vi "Edgertronic-get_camstatus.vi"(3 "error in (no error)":errorcluster, 5 "URL":string="192.168.1.101") -> (0 "error out":errorcluster, 1 "Cam Status":T2={"Level"="20140911165611", "Flags"="20140911165611", "Is Temp"="20140911165611", "FPGA Temp"="20140911165611", "State"="20140911165611", "Camera Time"="20140911165611", "dacvrefadc"="20140911165611", "Connection Information:"=""}, 2 "Status":T1={"Pretrigger Fill Level"=0, "IS Temp"=0.0, "State"=0, "dacvrefadc"="20140911165611", "Flags"={"Storage full"=FALSE, "Storage missing"=FALSE, "USB Storage installed"=FALSE, "SD Card installed"=FALSE, "USB full"=FALSE, "SD Card full"=FALSE, "Bad storage"=FALSE, "Net Configured"=FALSE, "Net unmountable"=FALSE, "Net full"=FALSE, "Storage full 11"=FALSE, "Storage full 12"=FALSE, "Storage full 13"=FALSE, "Storage full 14"=FALSE, "Storage full 15"=FALSE, "Storage full 16"=FALSE, "Storage full 17"=FALSE, "Genlock - no signal"=FALSE, "Genlock - config err"=FALSE}, "FPGA Temp"=0.0, "Camera time"=timestamp(0 s since 1904-01-01)} {"FPGA Temp" scale=0.0..100.0; "State" items=["Unconfigured", "Calibrating", "Running", "Triggered", "Saving", "Pretrigger full", "Trigger Canceled", "Save Canceled"]; "IS Temp" scale=0.0..100.0; "Pretrigger Fill Level" scale=0.0..100.0})   [LabVIEW 2015]
doc: "This VI returns the camera status information."
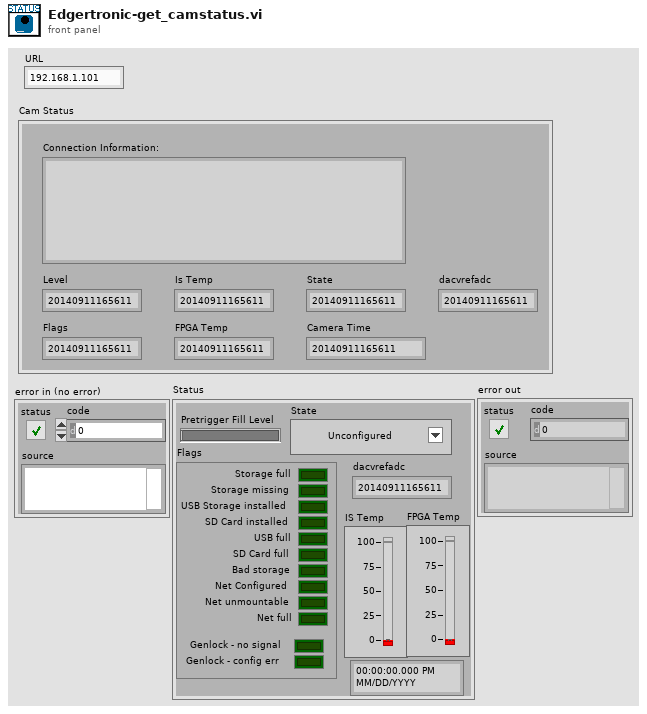
[diagram p1: front panel]
types:
  T1 = cluster{"Pretrigger Fill Level":u8, "IS Temp":dbl, "State":u16, "dacvrefadc":string, "Flags":cluster{"Storage full":bool, "Storage missing":bool, "USB Storage installed":bool, "SD Card installed":bool, "USB full":bool, "SD Card full":bool, "Bad storage":bool, "Net Configured":bool, "Net unmountable":bool, "Net full":bool, "Storage full 11":bool, "Storage full 12":bool, "Storage full 13":bool, "Storage full 14":bool, "Storage full 15":bool, "Storage full 16":bool, "Storage full 17":bool, "Genlock - no signal":bool, "Genlock - config err":bool}, "FPGA Temp":dbl, "Camera time":timestamp}
  T2 = cluster{"Level":string, "Flags":string, "Is Temp":string, "FPGA Temp":string, "State":string, "Camera Time":string, "dacvrefadc":string, "Connection Information:":string}
  T3 = cluster{"Boolean array[0]":bool, "Boolean array[1]":bool, "Boolean array[2]":bool, "Boolean array[3]":bool, "Boolean array[4]":bool, "Boolean array[5]":bool, "Boolean array[6]":bool, "Boolean array[7]":bool, "Boolean array[8]":bool, "Boolean array[9]":bool, "Boolean array[10]":bool, "Boolean array[11]":bool, "Boolean array[12]":bool, "Boolean array[13]":bool, "Boolean array[14]":bool, "Boolean array[15]":bool, "Boolean array[16]":bool, "Boolean array[17]":bool, "Boolean array[18]":bool}
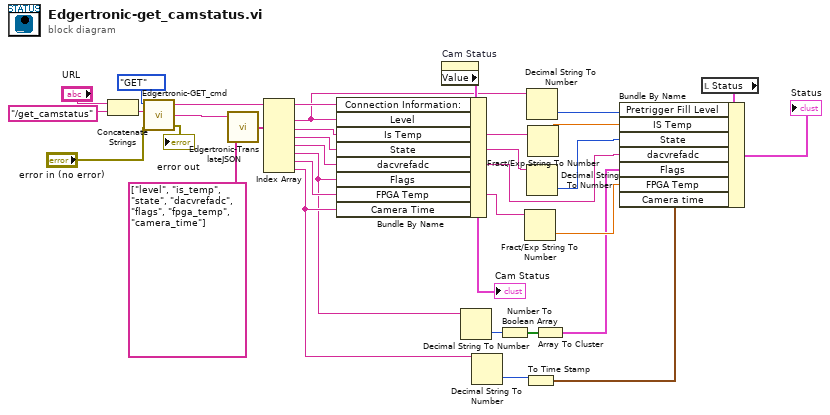
[diagram p0: block diagram]
diagram:
  n1 = Concatenate Strings("URL", "/get_camstatus" ("GET Cmd")) -> (w3:string)
  n2 = call "Edgertronic-GET_cmd.vi"("error in (no error)"="error in (no error)", "URL"=w3, "Type"=enum16{"GET", "POST"}."GET") -> ("error out"=→"error out":errorcluster, "data"=w27:string, "Connection Info"=w28:string)  [unwired: 1 in]
  n3 = call "Edgertronic-TranslateJSON.vi"("Commands"=string[] ["level", "is_temp", "state", "dacvrefadc", "flags", "fpga_temp", "camera_time"], "data"=w27) -> ("Values"=w25:string[])  [unwired: 3 in]
  n4 = Index Array(array=w25) -> (element #1=w21:string, element #2=w19:string, element #3=w17:string, element #4=w15:string, element #5=w7:string, element #6=w14:string, element #7=w12:string)  [unwired: 7 in]
  n5 = property on="Cam Status" class="Clust (strict)"() -> ("Value"=w26:T2)  [unwired: 2 in, 2 out]
  n6 = Bundle By Name(cluster=w26, "Connection Information:"=w28, "Level"=w21, "Is Temp"=w19, "State"=w17, "dacvrefadc"=w15, "Flags"=w7, "FPGA Temp"=w14, "Camera Time"=w12) -> (→"Cam Status":T2)
  n7 = Decimal String To Number(string=w7) -> (number=w8:i32)  [unwired: 2 in, 1 out]
  n8 = Decimal String To Number(string=w12) -> (number=w11:i32)  [unwired: 2 in, 1 out]
  n9 = Number To Boolean Array(number=w8) -> (Boolean array=w9:bool[])
  n10 = Fract/Exp String To Number(string=w14) -> (number=w13:dbl)  [unwired: 3 in, 1 out]
  n11 = To Time Stamp(1:w11) -> (0:w10:timestamp)
  n12 = Decimal String To Number(string=w21) -> (number=w20:i32)  [unwired: 2 in, 1 out]
  n13 = Decimal String To Number(string=w17) -> (number=w16:i32)  [unwired: 2 in, 1 out]
  n14 = Fract/Exp String To Number(string=w19) -> (number=w18:dbl)  [unwired: 3 in, 1 out]
  n15 = Array To Cluster(array=w9) -> (cluster=w6:T3)
  n16 = local read "Status"() -> (w23:T1)
  n17 = Bundle By Name(cluster=w23, "Pretrigger Fill Level"=w20, "IS Temp"=w18, "State"=w16, "dacvrefadc"=w15, "Flags"=w6, "FPGA Temp"=w13, "Camera time"=w10) -> (→"Status":T1)
